vi "StateSpaceUtil_PoseTo4dVector.vi"(11 "Pose":T2={"TRANSLATION"={"X"=0.0, "Y"=0.0}, "ROTATION"={"VALUE"=0.0, "COS"=1.0, "SIN"=0.0}} {"ROTATION"."SIN" format="%13.4f"; "ROTATION"."COS" format="%13.4f"; "ROTATION"."VALUE" format="%13.4f"; "TRANSLATION"."Y" format="%14.3f"; "TRANSLATION"."X" format="%14.3f"}) -> (3 "Pose Vector":T1)   [LabVIEW 2019, in "Trajectory_Library.lvlib"]
doc: "Creates a new LINEAR SYSTEM data cluster with the specified values. \n\n\nInputs: \n - XXX -- XXX.\n\nOutputs:\n - XXX -- XXX."
uses:
  POSE2D.ctl
  TRANSLATION2D.ctl
  ROTATION2D.ctl
  <vilib>/Analysis/Matrix/Datatypes/RealMatrix.ctl
  MatBuilder_Create.vi
  Trajectory_Library.lvlib
  <vilib>/Analysis/Matrix/NI_Matrix.lvlib
panel:
  # "<4, 1>"
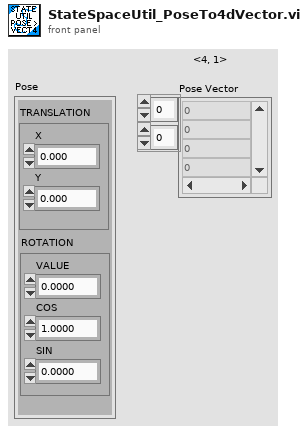
[diagram p1: front panel]
types:
  T1 = typedef "NI_Matrix.lvlib/RealMatrix.ctl" = dbl[][]
  T2 = typedef "Trajectory_Library.lvlib/POSE2D.ctl" = cluster{"TRANSLATION":T3, "ROTATION":T4}
  T3 = typedef "Trajectory_Library.lvlib/TRANSLATION2D.ctl" = cluster{"X":dbl, "Y":dbl}
  T4 = typedef "Trajectory_Library.lvlib/ROTATION2D.ctl" = cluster{"VALUE":dbl, "COS":dbl, "SIN":dbl}
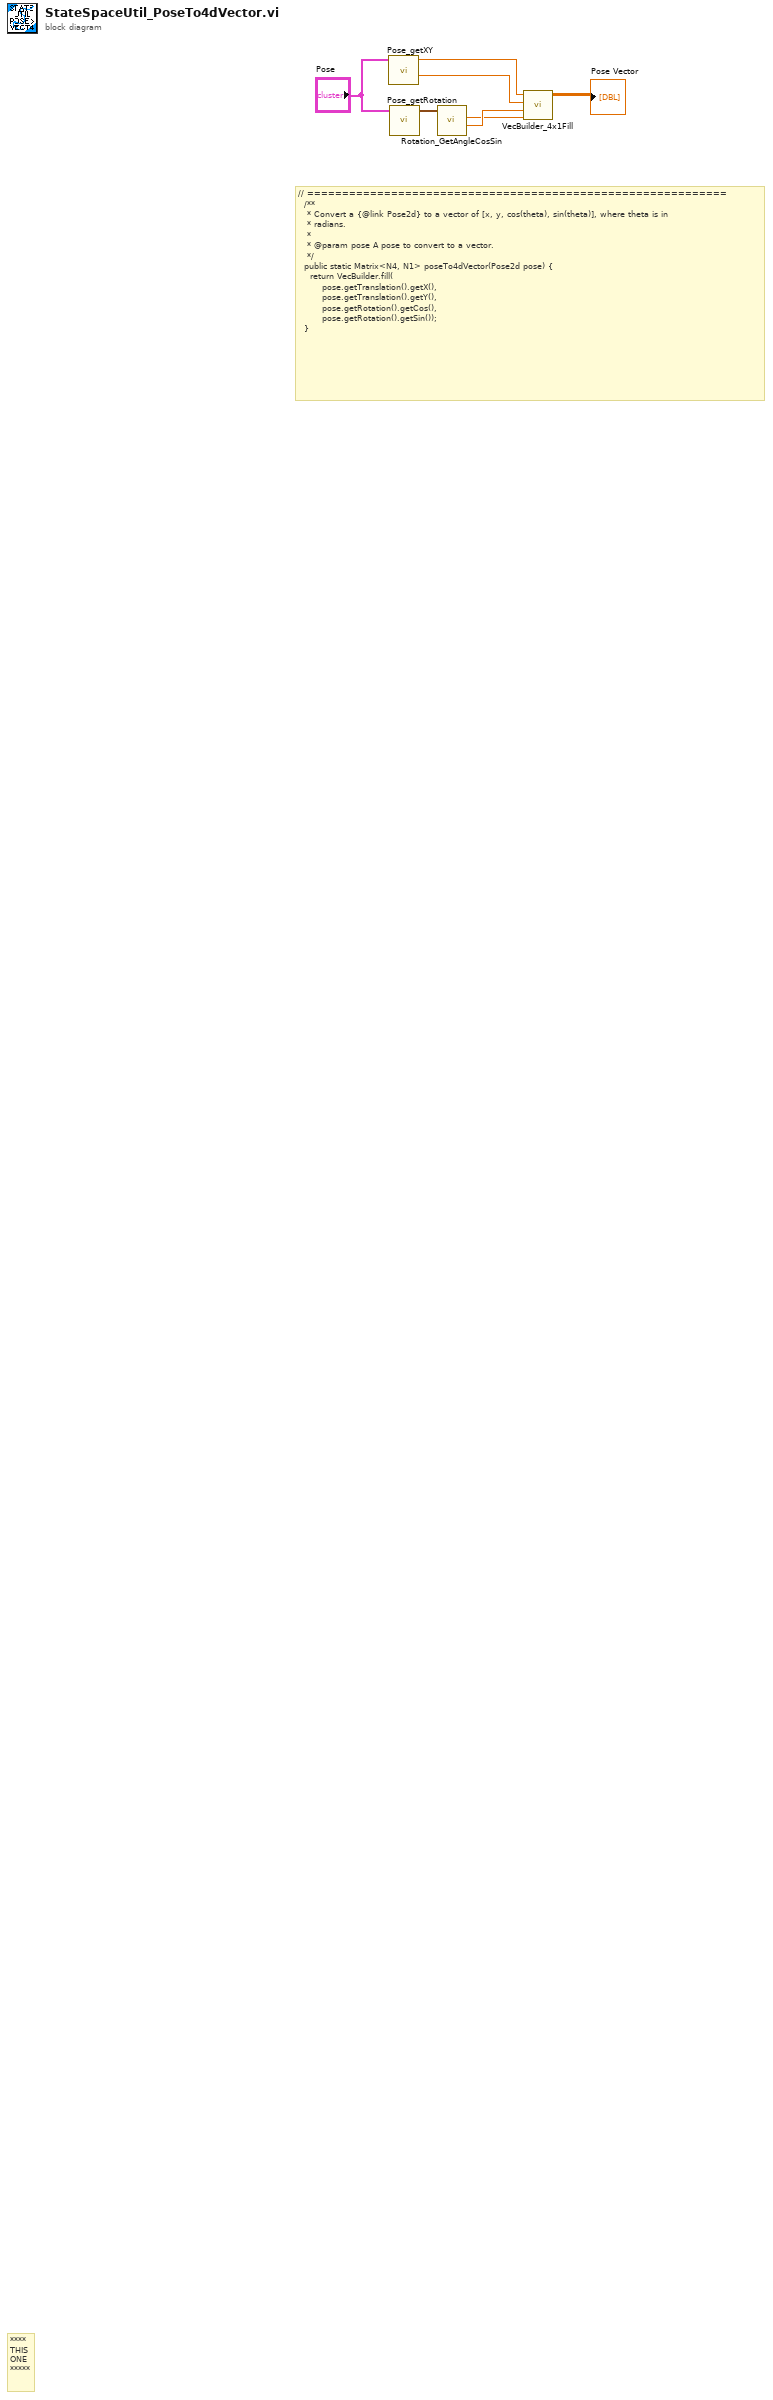
[diagram p0: block diagram]
diagram:
  # "// ============================================================\n  /**\n   * Convert a {@link Pose2d} to a vector of [x, y, cos(theta), sin(theta)], where theta is in\n   * radians.\n   *\n   * @param pose A pose to convert to a vector.\n   */\n  public static Matrix<N4, N1> poseTo4dVector(Pose2d pose) {\n    return VecBuilder.fill(\n        pose.getTranslation().getX(),\n        pose.getTranslation().getY(),\n        pose.getRotation().getCos(),\n        pose.getRotation().getSin());\n  }"
  # "****\nTHIS\nONE\n*****"
  n1 = call "Pose_getXY.vi"("in POSE"="Pose") -> ("Y"=w3:dbl, "X"=w4:dbl)  [unwired: 9 in]
  n2 = call "Pose_getRotation.vi"("in POSE"="Pose") -> ("out ROTATION"=w6:T4)  [unwired: 10 in]
  n3 = call "Rotation_GetAngleCosSin.vi"("in ROTATION"=w6) -> ("Cosine"=w2:dbl, "Sine"=w1:dbl)  [unwired: 8 in, 1 out]
  n4 = call "VecBuilder_4x1Fill.vi"("R3"=w1, "R2"=w2, "R1"=w3, "R0"=w4) -> ("output matrix"=→"Pose Vector":T1)  [unwired: 7 in]
